vi "sub_GSlam_calc-rotational-matrix.vi"() -> ()   [LabVIEW 2019]
uses:
  <vilib>/Analysis/coordinate.llb/Euler Rotation Order.ctl
  <vilib>/Analysis/NI_AALPro.lvlib
panel:
  out "Direction Cosines":dbl[][](array[numeric]) caption="방향 코사인"
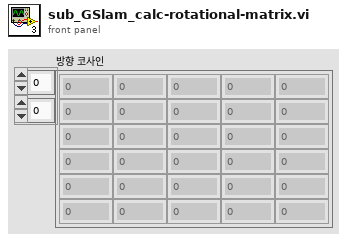
[diagram p1: front panel]
types:
  T1 = typedef "NI_AALPro.lvlib/Euler Rotation Order.ctl" = u16
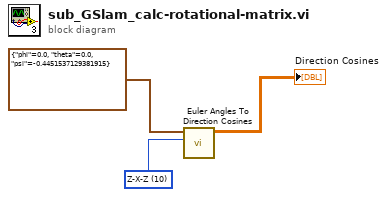
[diagram p0: block diagram]
diagram:
  w2 = T1 10 items=["X-Y-Z", "X-Z-Y", "Y-X-Z", "Y-Z-X", "Z-X-Y", "Z-Y-X", "X-Y-X", "X-Z-X", "Y-X-Y", "Y-Z-Y", "Z-X-Z", "Z-Y-Z"] ("rotation order")
  n1 = call <vilib>:"Euler Angles To Direction Cosines.vi"("rotation order"=w2, "Euler Angles"=cluster{"phi":dbl, "theta":dbl, "psi":dbl} {"phi"=0.0, "theta"=0.0, "psi"=-0.4451537129381915}) -> ("Direction Cosines"=→"Direction Cosines":dbl[][])  [unwired: 8 in, 1 out]
